vi "DB_query.vi"(11 "Humidity":string) -> (3 "String":string)   [LabVIEW 2018]
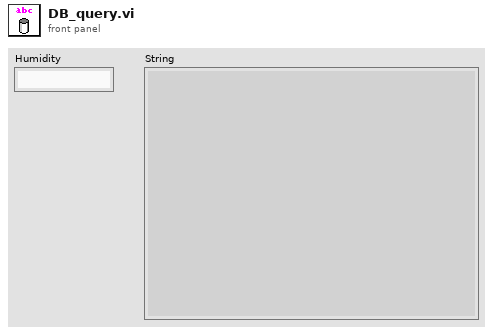
[diagram p1: front panel]
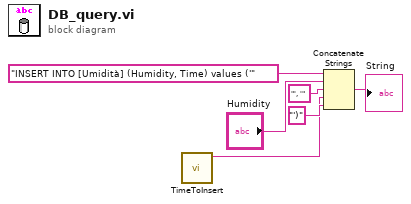
[diagram p0: block diagram]
diagram:
  n1 = call "TimeToInsert.vi"() -> ("Time"=w5:string)  [unwired: 11 in]
  n2 = Concatenate Strings("INSERT INTO [Umidità] (Humidity, Time) values ('" ("string"), "Humidity", "', '" ("string"), w5, "')" ("string")) -> (→"String":string)
